vi "KE2260B VI Tree.vi"   [LabVIEW 2009, in "Keithley 2260B.lvlib"]
doc: "This is the instrument driver for the <INSTRUMENT NAME>. The VI Tree displays all the user-callable VIs of the instrument driver in an organized table."
uses:
  <instrlib>/Keithley 2260B/Keithley 2260B.lvlib
panel:
  # "SEE DIAGRAM\nFOR VI TREE."
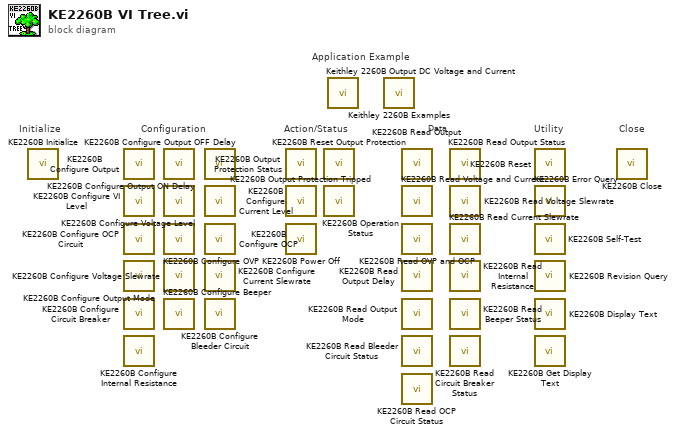
[diagram p0: block diagram]
diagram:
  # "Application Example"
  # "Configuration"
  # "Utility"
  # "Data"
  # "Action/Status"
  # "Close"
  # "Initialize"
  n1 = call <instrlib>:"KE2260B Initialize.vi"() -> ()  [unwired: 10 in, 2 out]
  n2 = call <instrlib>:"KE2260B Configure Output.vi"() -> ()  [unwired: 10 in, 2 out]
  n3 = call <instrlib>:"KE2260B Configure VI Level.vi"() -> ()  [unwired: 10 in, 2 out]
  n4 = call <instrlib>:"KE2260B Configure OCP Circuit.vi"() -> ()  [unwired: 10 in, 2 out]
  n5 = call <instrlib>:"KE2260B Configure Output Mode.vi"() -> ()  [unwired: 10 in, 2 out]
  n6 = call <instrlib>:"KE2260B Configure Circuit Breaker.vi"() -> ()  [unwired: 10 in, 2 out]
  n7 = call <instrlib>:"KE2260B Configure Internal Resistance.vi"() -> ()  [unwired: 10 in, 2 out]
  n8 = call <instrlib>:"KE2260B Configure Output ON Delay.vi"() -> ()  [unwired: 10 in, 2 out]
  n9 = call <instrlib>:"KE2260B Configure Voltage Level.vi"() -> ()  [unwired: 10 in, 2 out]
  n10 = call <instrlib>:"KE2260B Configure OVP.vi"() -> ()  [unwired: 10 in, 2 out]
  n11 = call <instrlib>:"KE2260B Configure Voltage Slewrate.vi"() -> ()  [unwired: 10 in, 2 out]
  n12 = call <instrlib>:"KE2260B Configure Beeper.vi"() -> ()  [unwired: 10 in, 2 out]
  n13 = call <instrlib>:"KE2260B Configure Output OFF Delay.vi"() -> ()  [unwired: 10 in, 2 out]
  n14 = call <instrlib>:"KE2260B Configure Current Level.vi"() -> ()  [unwired: 10 in, 2 out]
  n15 = call <instrlib>:"KE2260B Configure OCP.vi"() -> ()  [unwired: 10 in, 2 out]
  n16 = call <instrlib>:"KE2260B Configure Current Slewrate.vi"() -> ()  [unwired: 10 in, 2 out]
  n17 = call <instrlib>:"KE2260B Configure Bleeder Circuit.vi"() -> ()  [unwired: 10 in, 2 out]
  n18 = call <instrlib>:"KE2260B Output Protection Status.vi"() -> ()  [unwired: 8 in, 4 out]
  n19 = call <instrlib>:"KE2260B Output Protection Tripped.vi"() -> ()  [unwired: 4 in, 8 out]
  n20 = call <instrlib>:"KE2260B Power Off.vi"() -> ()  [unwired: 10 in, 2 out]
  n21 = call <instrlib>:"KE2260B Reset Output Protection.vi"() -> ()  [unwired: 10 in, 2 out]
  n22 = call <instrlib>:"KE2260B Operation Status.vi"() -> ()  [unwired: 6 in, 6 out]
  n23 = call <instrlib>:"Keithley 2260B Output DC Voltage and Current.vi"() -> ()  [unwired: 12 in]
  n24 = call <instrlib>:"Keithley 2260B Examples.vi"() -> ()  [unwired: 12 in]
  n25 = call <instrlib>:"KE2260B Read Output.vi"() -> ()  [unwired: 8 in, 4 out]
  n26 = call <instrlib>:"KE2260B Read Voltage and Current.vi"() -> ()  [unwired: 8 in, 4 out]
  n27 = call <instrlib>:"KE2260B Read OVP and OCP.vi"() -> ()  [unwired: 8 in, 4 out]
  n28 = call <instrlib>:"KE2260B Read Output Delay.vi"() -> ()  [unwired: 8 in, 4 out]
  n29 = call <instrlib>:"KE2260B Read Output Mode.vi"() -> ()  [unwired: 9 in, 3 out]
  n30 = call <instrlib>:"KE2260B Read Bleeder Circuit Status.vi"() -> ()  [unwired: 9 in, 3 out]
  n31 = call <instrlib>:"KE2260B Read OCP Circuit Status.vi"() -> ()  [unwired: 9 in, 3 out]
  n32 = call <instrlib>:"KE2260B Read Output Status.vi"() -> ()  [unwired: 9 in, 3 out]
  n33 = call <instrlib>:"KE2260B Read Voltage Slewrate.vi"() -> ()  [unwired: 8 in, 4 out]
  n34 = call <instrlib>:"KE2260B Read Current Slewrate.vi"() -> ()  [unwired: 8 in, 4 out]
  n35 = call <instrlib>:"KE2260B Read Internal Resistance.vi"() -> ()  [unwired: 9 in, 3 out]
  n36 = call <instrlib>:"KE2260B Read Beeper Status.vi"() -> ()  [unwired: 9 in, 3 out]
  n37 = call <instrlib>:"KE2260B Read Circuit Breaker Status.vi"() -> ()  [unwired: 9 in, 3 out]
  n38 = call <instrlib>:"KE2260B Reset.vi"() -> ()  [unwired: 10 in, 2 out]
  n39 = call <instrlib>:"KE2260B Error Query.vi"() -> ()  [unwired: 8 in, 4 out]
  n40 = call <instrlib>:"KE2260B Self-Test.vi"() -> ()  [unwired: 8 in, 4 out]
  n41 = call <instrlib>:"KE2260B Revision Query.vi"() -> ()  [unwired: 8 in, 4 out]
  n42 = call <instrlib>:"KE2260B Display Text.vi"() -> ()  [unwired: 10 in, 2 out]
  n43 = call <instrlib>:"KE2260B Get Display Text.vi"() -> ()  [unwired: 7 in, 5 out]
  n44 = call <instrlib>:"KE2260B Close.vi"() -> ()  [unwired: 11 in, 1 out]
